vi "Measurement Query.vi"(0 "Instrument Handle In":i32, 5 "error in":errorcluster) -> (6 "High Reference":dbl, 7 "Edge Number":i32, 8 "Mid Reference":dbl, 9 "Gate Stop Freq":dbl caption="Gate Stop Frequency", 10 "Low Reference":dbl, 11 "Gate Start Freq":dbl caption="Gate Start Frequency", 12 "Reference Method":i32, 13 "Gate Stop Points":u32, 14 "Instrument Handle Out":i32, 15 "Method":i32, 16 "Gate Start Time":dbl, 17 "Gate Stop Time":dbl, 18 "Gate Start Points":u32, 19 "error out":errorcluster)   [LabVIEW 8.6, in "ZTScopeM.lvlib"]
doc: "Query the measurement settings"
uses:
  ZTScopeM.lvlib
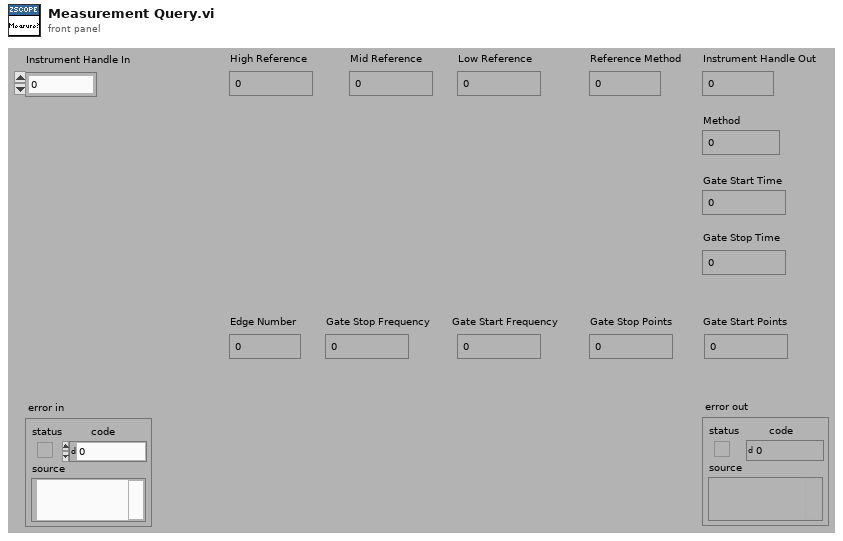
[diagram p1: front panel]
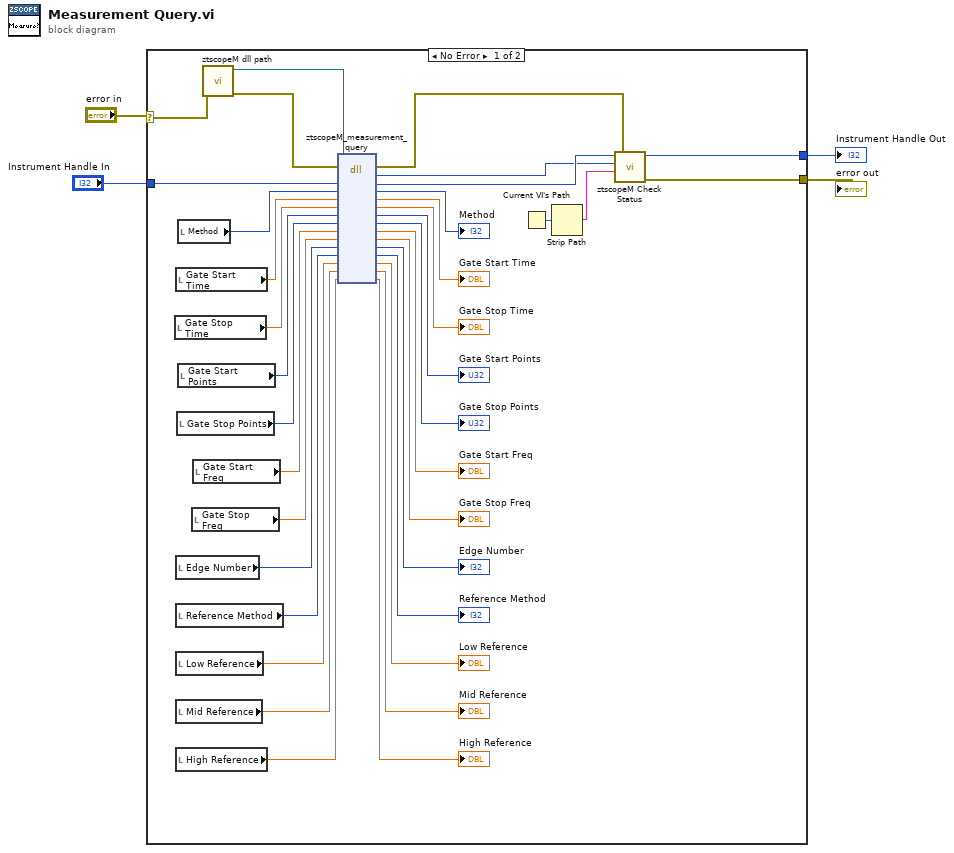
[diagram p0: block diagram]
diagram:
  n1 = case shown="No Error" "error in" {
    selector: "error in" -> [w8 w41]
    tunnel: [w10 w41] -> w2
    tunnel: "Instrument Handle In" -> [w39 w40]
    tunnel: [w9 w40] -> w3
    frame #0 {
      n2 = local read "Gate Stop Time"() -> (w34:dbl)
      n3 = local read "Gate Start Time"() -> (w36:dbl)
      n4 = local read "Edge Number"() -> (w24:i32)
      n5 = local read "Reference Method"() -> (w22:i32)
      n6 = local read "Low Reference"() -> (w20:dbl)
      n7 = local read "Mid Reference"() -> (w18:dbl)
      n8 = local read "High Reference"() -> (w16:dbl)
      n9 = local read "Gate Stop Points"() -> (w30:u32)
      n10 = local read "Method"() -> (w38:i32)
      n11 = local read "Gate Start Points"() -> (w32:u32)
      n12 = local read "Gate Stop Freq"() -> (w26:dbl)
      n13 = local read "Gate Start Freq"() -> (w28:dbl)
      n14 = call "ztscopeM dll path.vi"("error in (no error)"=w8) -> ("error out"=w6:errorcluster, "<instrument>.dll path"=w7:path)  [unwired: 9 in]
      n15 = dll-call lib="C:/Program Files (x86)/National Instruments/LabVIEW 2013/instr.lib/ztscopem/ztscopeM.dll" fn="ztscopeM_measurement_query"(path in=w7, error in=w6, "instrumentHandle"=w39, "method"=w38, "gateStartTime"=w36, "gateStopTime"=w34, "gateStartPoints"=w32, "gateStopPoints"=w30, "gateStartFrequency"=w28, "gateStopFrequency"=w26, "edgeNumber"=w24, "referenceMethod"=w22, "lowReference"=w20, "midReference"=w18, "highReference"=w16) -> (error out=w5:errorcluster, w11:i32, "instrumentHandle"=w12:i32, "method"=→"Method":i32, "gateStartTime"=→"Gate Start Time":dbl, "gateStopTime"=→"Gate Stop Time":dbl, "gateStartPoints"=→"Gate Start Points":u32, "gateStopPoints"=→"Gate Stop Points":u32, "gateStartFrequency"=→"Gate Start Freq":dbl, "gateStopFrequency"=→"Gate Stop Freq":dbl, "edgeNumber"=→"Edge Number":i32, "referenceMethod"=→"Reference Method":i32, "lowReference"=→"Low Reference":dbl, "midReference"=→"Mid Reference":dbl, "highReference"=→"High Reference":dbl)  [unwired: 1 in, 1 out]
      n16 = Current VI's Path() -> (path=w14:path)
      n17 = Strip Path(path=w14) -> (name=w13:string)  [unwired: 1 out]
      n18 = call "ztscopeM Check Status.vi"("error in"=w5, "name of VI"=w13, "status (return code)"=w11, "instrument handle in"=w12) -> ("error out"=w10:errorcluster, "instrument handle out"=w9:i32)  [unwired: 2 in]
    }
    frame #1 {
    }
  }
  "Instrument Handle Out" <- w3
  "error out" <- w2
